vi "Save Network Settings.vi"(8 "error in (no error)":errorcluster, 11 "VISA resource name":refnum<visa-resource-name>) -> (0 "error out":errorcluster, 3 "VISA resource name out":refnum<visa-resource-name>)   [LabVIEW 2013, in "Watts Up PRO Net Series.lvlib"]
doc: "Saves the current set network/internet configurations to non-volatile memory so that the configurations can be retrieved during a power off of the Watts Up .Net device."
uses:
  <instrlib>/Watts Up PRO Net Series/Watts Up PRO Net Series.lvlib
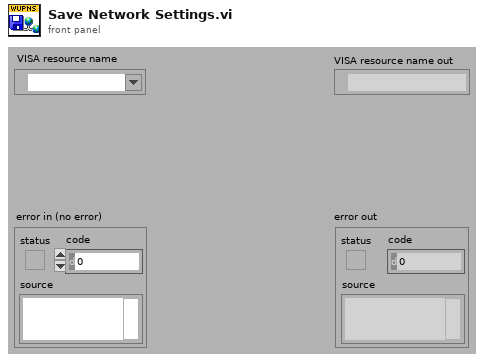
[diagram p1: front panel]
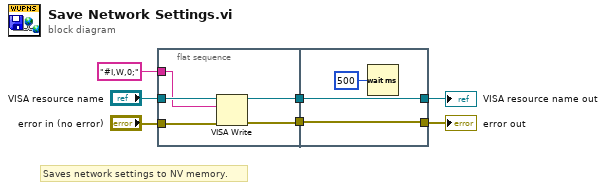
[diagram p0: block diagram]
diagram:
  # "Saves network settings to NV memory."
  n1 = flat-sequence {
    tunnel: "VISA resource name" -> [w12]
    tunnel: "error in (no error)" -> [w11]
    tunnel: "#I,W,0;" ("write buffer") -> [w8]
    tunnel: [w10] -> w2
    tunnel: [w9] -> w1
    tunnel: [w14] -> w4
    tunnel: [w15] -> w5
    tunnel: w2 -> [w15]
    tunnel: w1 -> [w14]
    frame #0 {
      n2 = VISA Write(VISA resource name=w12, write buffer=w8, error in (no error)=w11) -> (VISA resource name out=w10:refnum<visa-resource-name>, error out=w9:errorcluster)  [unwired: 1 out]
    }
    frame #1 {
      n3 = Wait (ms)(milliseconds to wait=u32 500) -> ()  [unwired: 1 out]
    }
  }
  "VISA resource name out" <- w5
  "error out" <- w4
